vi "AndOr.vi"(9 "Teams in":i32[][](array[numeric]), 10 "AndOr1":enum16{"And", "Or"}(ring)=enum."Or", 11 "AndOr2":enum16{"And", "Or"}(ring)=enum."Or") -> (3 "Teams out":i32[](array[numeric]))   [LabVIEW 2017]
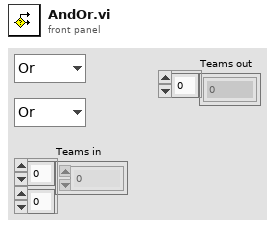
[diagram p1: front panel]
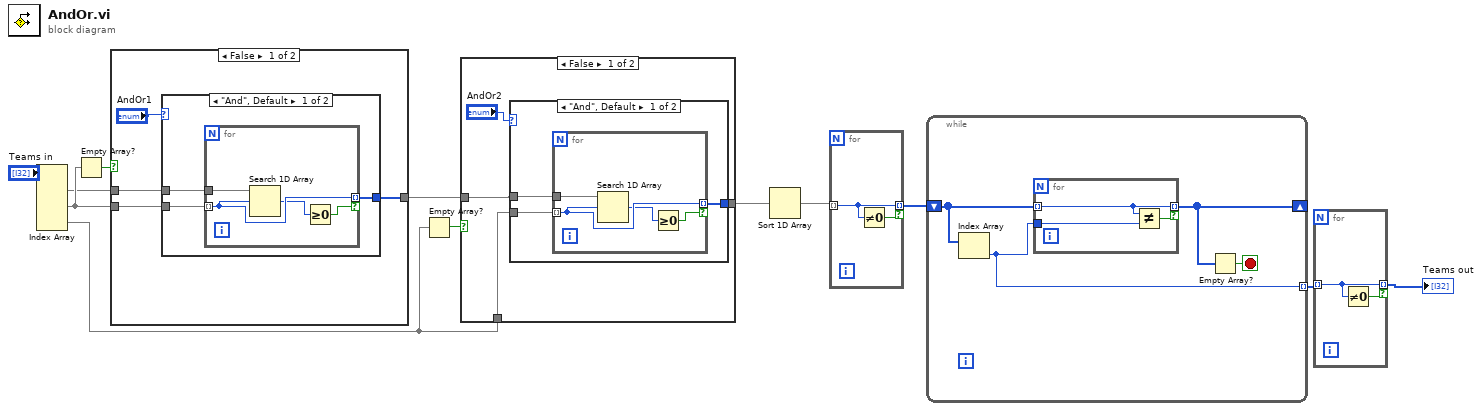
[diagram p0: block diagram]
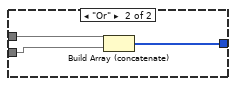
[diagram p2: hidden frame]
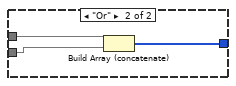
[diagram p4: hidden frame]
diagram:
  n1 = Index Array(array="Teams in") -> (element #1=w6:i32[], element #2=w9:i32[], element #3=w11:i32[])  [unwired: 6 in]
  n2 = Empty Array?(array=w9) -> (empty?=w10:bool)
  n3 = case shown="False" w10 {
    tunnel: w6 -> [w15 w27]
    tunnel: [w14 w27] -> w7
    tunnel: w9 -> [w13 _]
    frame False {
      n4 = case shown="\"And\", Default" "AndOr1" {
        tunnel: w13 -> [w18 w26]
        tunnel: w15 -> [w19 w25]
        tunnel: [w17 w24] -> w14
        frame "And", Default {
          n5 = for {
            tunnel: w19 -> [w23]
            tunnel: w18 -> [w22] mode=indexing
            tunnel: [w22] -> w17 mode=indexing if=w21
            n6 = Search 1D Array(1D array=w23, element=w22) -> (index of element=w20:i32)  [unwired: 1 in]
            n7 = Greater Or Equal To 0?(x=w20) -> (x >= 0?=w21:bool)
          }
        }
        frame "Or" {
          n8 = Build Array (concatenate)(w25, w26) -> (w24:i32[])
        }
      }
    }
    frame True {
    }
  }
  n9 = Empty Array?(array=w11) -> (empty?=w12:bool)
  n10 = case shown="False" w12 {
    tunnel: w7 -> [w31 w42]
    tunnel: [w30 w42] -> w8
    tunnel: w11 -> [w28 _]
    frame False {
      n11 = case shown="\"And\", Default" "AndOr2" {
        tunnel: w28 -> [w33 w41]
        tunnel: w31 -> [w34 w40]
        tunnel: [w32 w39] -> w30
        frame "And", Default {
          n12 = for {
            tunnel: w34 -> [w38]
            tunnel: w33 -> [w37] mode=indexing
            tunnel: [w37] -> w32 mode=indexing if=w36
            n13 = Search 1D Array(1D array=w38, element=w37) -> (index of element=w35:i32)  [unwired: 1 in]
            n14 = Greater Or Equal To 0?(x=w35) -> (x >= 0?=w36:bool)
          }
        }
        frame "Or" {
          n15 = Build Array (concatenate)(w40, w41) -> (w39:i32[])
        }
      }
    }
    frame True {
    }
  }
  n16 = Sort 1D Array(array=w8) -> (sorted array=w3:i32[])
  n17 = for {
    tunnel: [w43] -> w4 mode=indexing if=w44
    tunnel: w3 -> [w43] mode=indexing
    n18 = Not Equal To 0?(x=w43) -> (x != 0?=w44:bool)
  }
  n19 = while {
    shift-right: [w46] -> _
    shift-left: w4 -> [w48]
    tunnel: [w47] -> w2 mode=indexing
    stop <- w45 stop-if-true
    n20 = Index Array(array=w48) -> (element=w47:i32)  [unwired: 1 in]
    n21 = for {
      tunnel: [w50] -> w46 mode=indexing if=w51
      tunnel: w48 -> [w50] mode=indexing
      tunnel: w47 -> [w49]
      n22 = Not Equal?(x=w50, y=w49) -> (x != y?=w51:bool)
    }
    n23 = Empty Array?(array=w46) -> (empty?=w45:bool)
  }
  n24 = for {
    tunnel: [w52] -> w1 mode=indexing if=w53
    tunnel: w2 -> [w52] mode=indexing
    n25 = Not Equal To 0?(x=w52) -> (x != 0?=w53:bool)
  }
  "Teams out" <- w1
